vi "RelativeMoveChannelsList.vi"() -> (3 "RelativeMoveChannels[]":string[](array[string]))   [LabVIEW 2013]
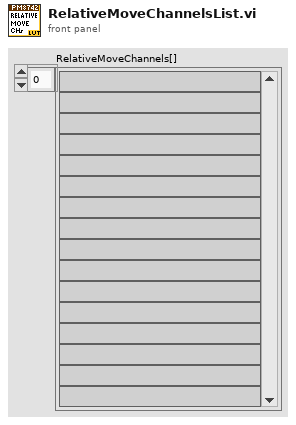
[diagram p1: front panel]
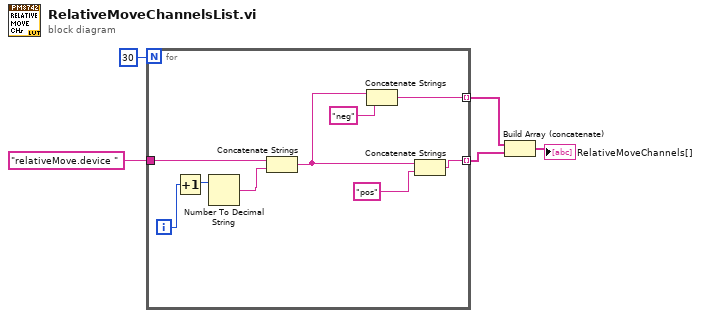
[diagram p0: block diagram]
diagram:
  n1 = for {
    N: 30 -> [_]
    tunnel: "relativeMove.device " -> [w12]
    tunnel: [w9] -> w4 mode=indexing
    tunnel: [w8] -> w5 mode=indexing
    i -> [w13]
    n2 = Increment(x=w13) -> (x+1=w14:i32)
    n3 = Number To Decimal String(number=w14) -> (decimal integer string=w7:string)  [unwired: 1 in]
    n4 = Concatenate Strings(w12, w7) -> (w6:string)
    n5 = Concatenate Strings(w6, "neg") -> (w9:string)
    n6 = Concatenate Strings(w6, "pos") -> (w8:string)
  }
  n7 = Build Array (concatenate)(w4, w5) -> (→"RelativeMoveChannels[]":string[])
